vi "例5.7“创建数组”函数.vi"() -> ()   [LabVIEW 2017]
panel:
  out "新数组（未选“连接输入”）":i32[][](array[numeric])
  out "新数组（选择“连接输入”）":i32[](array[numeric])
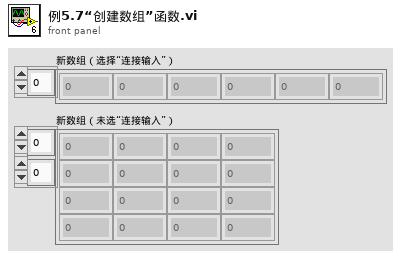
[diagram p1: front panel]
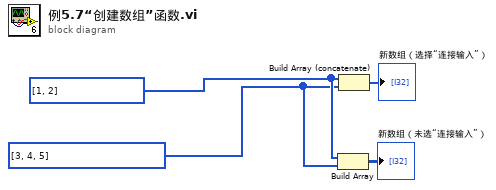
[diagram p0: block diagram]
diagram:
  w3 = i32[] [3, 4, 5]
  w4 = i32[] [1, 2]
  n1 = Build Array(w4, w3) -> (→"新数组（未选“连接输入”）":i32[][])
  n2 = Build Array (concatenate)(w4, w3) -> (→"新数组（选择“连接输入”）":i32[])
